vi "Serialize Experimental Data.vi"(0 "Save Destination":path) -> ()   [LabVIEW 2013]
uses:
  Experiment Serialized Data.ctl
  <vilib>/Utility/xml.llb/Write to XML File(string).vi
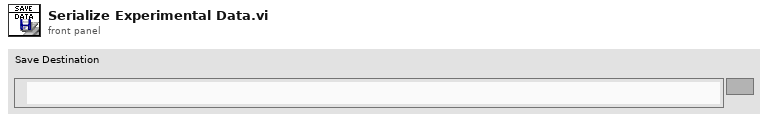
[diagram p1: front panel]
types:
  T1 = typedef "Experiment Serialized Data.ctl" = cluster{"Force Data":dbl[], "Signal Strength Data":dbl[], "X Position Data":dbl[], "Y Position Data":dbl[], "Z Position Data":dbl[], "Ramp Rate":dbl, "Z Scan Size":dbl, "Slope":dbl, "Spring Constant":dbl, string}
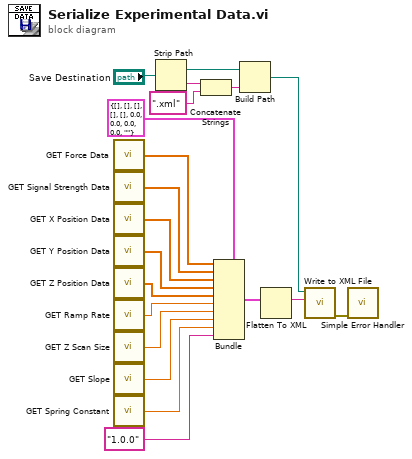
[diagram p0: block diagram]
diagram:
  n1 = call "GET Force Data.vi"() -> ("Force Data"=w14:dbl[])
  n2 = call "GET Signal Strength Data.vi"() -> ("Signal Strength Data"=w15:dbl[])
  n3 = call "GET X Position Data.vi"() -> ("X Position Data"=w16:dbl[])
  n4 = call "GET Y Position Data.vi"() -> ("Y Position Data"=w18:dbl[])
  n5 = call "GET Z Position Data.vi"() -> ("Z Position Data"=w20:dbl[])
  n6 = call "GET Ramp Rate.vi"() -> ("Ramp Rate"=w19:dbl)
  n7 = call "GET Z Scan Size.vi"() -> ("Z Scan Size"=w17:dbl)
  n8 = call "GET Slope.vi"() -> ("Slope"=w13:dbl)
  n9 = call "GET Spring Constant.vi"() -> ("Spring Constant"=w12:dbl)
  n10 = Strip Path(path="Save Destination") -> (stripped path=w2:path, name=w5:string)
  n11 = Concatenate Strings(w5, ".xml" ("string")) -> (w3:string)
  n12 = Bundle(cluster=T1 {"Force Data"=[], "Signal Strength Data"=[], "X Position Data"=[], "Y Position Data"=[], "Z Position Data"=[], "Ramp Rate"=0.0, "Z Scan Size"=0.0, "Slope"=0.0, "Spring Constant"=0.0, ""} ("Default Experiment Serialized Data"), "Force Data"=w14, "Signal Strength Data"=w15, "X Position Data"=w16, "Y Position Data"=w18, "Z Position Data"=w20, "Ramp Rate"=w19, "Z Scan Size"=w17, "Slope"=w13, "Spring Constant"=w12, "1.0.0") -> (w9:T1)
  n13 = Build Path(base path=w2, name or relative path=w3) -> (appended path=w1:path)
  n14 = Flatten To XML(anything=w9) -> (xml string=w8:string)
  n15 = call-poly <vilib>:"Write to XML File.vi"("XML Input"=w8, "XML File Path"=w1) -> ("error out"=w7:errorcluster)  [unwired: 7 in, 2 out]
  n16 = call <vilib>:"Simple Error Handler.vi"("error in (no error)"=w7) -> ()  [unwired: 4 in, 5 out]
